vi "Intake Get Sensors.vi"(1 "Intake Info In":T1) -> (0 "Intake Info In":T1)   [LabVIEW 2013]
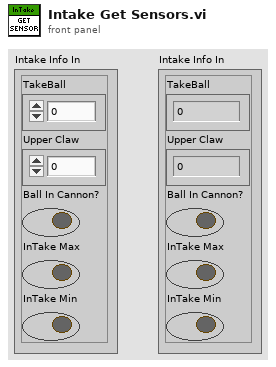
[diagram p1: front panel]
types:
  T1 = cluster{"TakeBall":dbl, "Upper Claw":dbl, "Ball In Cannon?":bool, "InTake Max":bool, "InTake Min":bool}
  T2 = typedef "WPI_DigitalInputDevRef.ctl" = cluster{"DevStatus":errorcluster, "DIO Channel":T3, "Digital Module":T4}
  T3 = typedef "FPGA_DIOChannel.ctl" = enum8{"DIO 1", "DIO 2", "DIO 3", "DIO 4", "DIO 5", "DIO 6", "DIO 7", "DIO 8", "DIO 9", "DIO 10", "DIO 11", "DIO 12", "DIO 13", "DIO 14", "Invalid"}
  T4 = typedef "FPGA_TypedefDigitalModule.ctl" = enum16{"Digital Module 1", "Digital Module 2"}
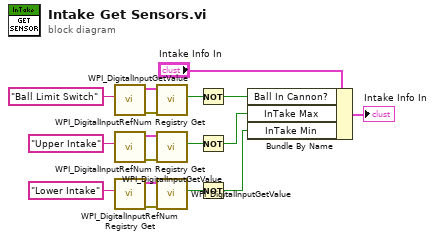
[diagram p0: block diagram]
diagram:
  n1 = call <vilib>:"WPI_DigitalInputRefNum Registry Get.vi"("refnum name"="Ball Limit Switch") -> ("error out"=w10:errorcluster, "DigitalInputDevRef"=w11:T2)  [unwired: 9 in]
  n2 = call <vilib>:"WPI_DigitalInputRefNum Registry Get.vi"("refnum name"="Upper Intake") -> ("error out"=w15:errorcluster, "DigitalInputDevRef"=w16:T2)  [unwired: 9 in]
  n3 = call <vilib>:"WPI_DigitalInputRefNum Registry Get.vi"("refnum name"="Lower Intake") -> ("error out"=w12:errorcluster, "DigitalInputDevRef"=w13:T2)  [unwired: 9 in]
  n4 = call <vilib>:"WPI_DigitalInputGetValue.vi"("error in (no error)"=w10, "DigitalInputDevRef"=w11) -> ("Value"=w6:bool)  [unwired: 7 in, 2 out]
  n5 = call <vilib>:"WPI_DigitalInputGetValue.vi"("error in (no error)"=w15, "DigitalInputDevRef"=w16) -> ("Value"=w4:bool)  [unwired: 7 in, 2 out]
  n6 = call <vilib>:"WPI_DigitalInputGetValue.vi"("error in (no error)"=w12, "DigitalInputDevRef"=w13) -> ("Value"=w5:bool)  [unwired: 7 in, 2 out]
  n7 = Not(x=w6) -> (.not. x?=w3:bool)
  n8 = Not(x=w4) -> (.not. x?=w2:bool)
  n9 = Not(x=w5) -> (.not. x?=w1:bool)
  n10 = Bundle By Name(cluster="Intake Info In", "Ball In Cannon?"=w3, "InTake Max"=w2, "InTake Min"=w1) -> (→"Intake Info In":T1)
